vi "Action Dispatch.vi"(8 "error in (no error)":errorcluster, 10 "Actions":T1(array[cluster]), 11 "Motions in":refnum<class "Motions.lvclass">) -> (0 "error out":errorcluster, 3 "Motions out":refnum<class "Motions.lvclass">)   [LabVIEW 2016, in "Hardware.lvlib" / "Motions.lvlib" / "Motions.lvclass"]
uses:
  <userlib>/Common Components/Hardware/Abstract System/Motions/Motions/Motions.lvclass
  <userlib>/Common Components/Hardware/Abstract System/Motions/Motions/Data_Set Motion Status.ctl
  <userlib>/Common Components/Hardware/Abstract System/Motions/Motions/Data_Move.ctl
  <userlib>/Common Components/Hardware/Abstract System/Motions/Motions/Data_Index.ctl
  <userlib>/Common Components/Hardware/Abstract System/Motions/Motions/Data_Update History Dst Q.ctl
  <vilib>/Utility/error.llb/Error Cluster From Error Code.vi
  <vilib>/ErrorRing/Error Ring.xnode
  <vilib>/addons/_JKI.lib/Serialization/JSON/JKI JSON Serialization.lvlib
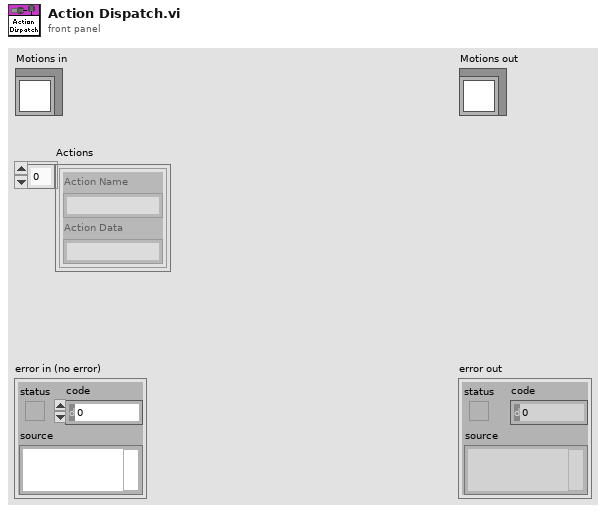
[diagram p1: front panel]
types:
  T1 = cluster{"Action Name":string, "Action Data":string}[]
  T2 = typedef "Hardware.lvlib/Motions.lvlib/Motions.lvclass/Data_Set Motion Status.ctl" = cluster{"Index":i32, "Motion Status":bool}
  T3 = typedef "Hardware.lvlib/Motions.lvlib/Motions.lvclass/Data_Move.ctl" = cluster{"Index":i32, "Destination":dbl}
  T4 = typedef "Hardware.lvlib/Motions.lvlib/Motions.lvclass/Data_Index.ctl" = cluster{"Index":i32}
  T5 = typedef "Hardware.lvlib/Motions.lvlib/Motions.lvclass/Data_Update History Dst Q.ctl" = cluster{"Index":i32, "Destination":dbl, "Mode":enum16{"Add", "Replace"}}
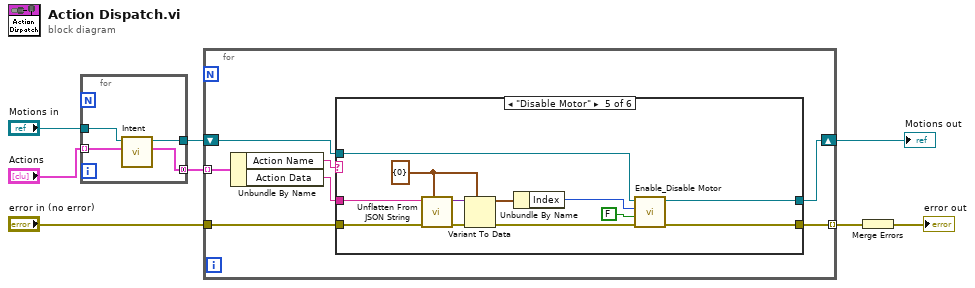
[diagram p0: block diagram]
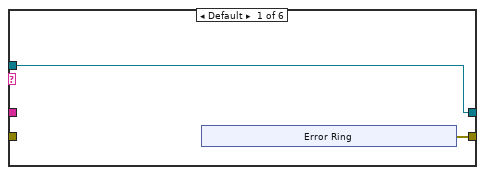
[diagram p2: hidden frame]
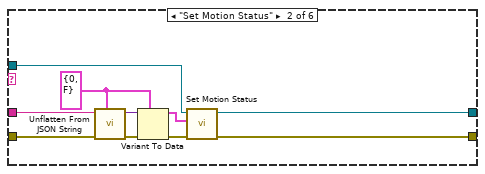
[diagram p3: hidden frame]
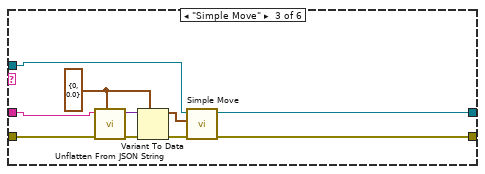
[diagram p4: hidden frame]
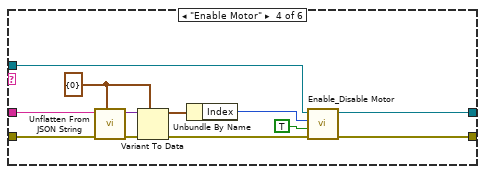
[diagram p5: hidden frame]
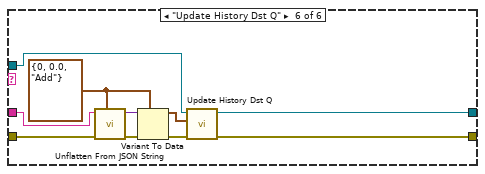
[diagram p6: hidden frame]
diagram:
  n1 = for {
    tunnel: "Actions" -> [w10] mode=indexing
    tunnel: "Motions in" -> [w12]
    tunnel: [w11] -> w2
    tunnel: [w9] -> w1 mode=concatenating
    n2 = call <userlib>:"Intent.vi"("Intent"=w10, "Motions in"=w12) -> ("Actions"=w9:T1, "Motions out"=w11:refnum<class "Motions.lvclass">)  [unwired: 7 in, 1 out]
  }
  n3 = for {
    shift-right: [w14] -> w8
    shift-left: w2 -> [w17]
    tunnel: w1 -> [w19] mode=indexing
    tunnel: "error in (no error)" -> [w15]
    tunnel: [w13] -> w6 mode=indexing
    n4 = Unbundle By Name(w19) -> ("Action Name"=w18:string, "Action Data"=w16:string)
    n5 = case shown="\"Disable Motor\"" w18 {
      tunnel: [w21 w26 w36 w50 w62 w79] -> w13
      tunnel: w17 -> [w20 w35 w40 w53 w65 w78]
      tunnel: w16 -> [_ w34 w41 w54 w66 w70]
      tunnel: w15 -> [_ w33 w43 w55 w67 w74]
      tunnel: [w20 w27 w37 w51 w63 w77] -> w14
      frame Default {
        n6 = xnode "Error Ring"() -> ("error out"=w21:errorcluster)
      }
      frame "Set Motion Status" {
        w31 = T2 {"Index"=0, "Motion Status"=FALSE} ("Set Motion Status Data cluster")
        n7 = call <vilib>:"Unflatten From JSON String.vi"("Type and Defaults"=w31, "error in (no error)"=w33, "JSON String"=w34) -> ("error out"=w30:errorcluster, "Variant"=w32:variant)  [unwired: 7 in]
        n8 = Variant To Data(error in=w30, type=w31, Variant=w32) -> (data=w28:T2, error out=w29:errorcluster)
        n9 = call <userlib>:"Set Motion Status.vi"("error in (no error)"=w29, "Set Motion Status Data cluster"=w28, "Motions in"=w35) -> ("error out"=w26:errorcluster, "Motions out"=w27:refnum<class "Motions.lvclass">)  [unwired: 7 in]
      }
      frame "Simple Move" {
        w42 = T3 {"Index"=0, "Destination"=0.0} ("Set Motion Status Data cluster")
        n10 = call <vilib>:"Unflatten From JSON String.vi"("Type and Defaults"=w42, "error in (no error)"=w43, "JSON String"=w41) -> ("error out"=w44:errorcluster, "Variant"=w45:variant)  [unwired: 7 in]
        n11 = Variant To Data(error in=w44, type=w42, Variant=w45) -> (data=w39:T3, error out=w38:errorcluster)
        n12 = call <userlib>:"Simple Move.vi"("error in (no error)"=w38, "Move Data cluster"=w39, "Motions in"=w40) -> ("error out"=w36:errorcluster, "Motions out"=w37:refnum<class "Motions.lvclass">)  [unwired: 7 in]
      }
      frame "Enable Motor" {
        w47 = T4 {"Index"=0} ("Move Data cluster")
        n13 = call <vilib>:"Unflatten From JSON String.vi"("Type and Defaults"=w47, "error in (no error)"=w55, "JSON String"=w54) -> ("error out"=w56:errorcluster, "Variant"=w57:variant)  [unwired: 7 in]
        n14 = Variant To Data(error in=w56, type=w47, Variant=w57) -> (data=w49:T4, error out=w52:errorcluster)
        n15 = Unbundle By Name(w49) -> ("Index"=w48:i32)
        n16 = call <userlib>:"Enable_Disable Motor.vi"("error in (no error)"=w52, "enable/disable"=TRUE, "Index"=w48, "Motions in"=w53) -> ("error out"=w50:errorcluster, "Motions out"=w51:refnum<class "Motions.lvclass">)  [unwired: 6 in]
      }
      frame "Disable Motor" {
        w59 = T4 {"Index"=0} ("Move Data cluster")
        n17 = call <vilib>:"Unflatten From JSON String.vi"("Type and Defaults"=w59, "error in (no error)"=w67, "JSON String"=w66) -> ("error out"=w68:errorcluster, "Variant"=w69:variant)  [unwired: 7 in]
        n18 = Variant To Data(error in=w68, type=w59, Variant=w69) -> (data=w61:T4, error out=w64:errorcluster)
        n19 = Unbundle By Name(w61) -> ("Index"=w60:i32)
        n20 = call <userlib>:"Enable_Disable Motor.vi"("error in (no error)"=w64, "enable/disable"=FALSE, "Index"=w60, "Motions in"=w65) -> ("error out"=w62:errorcluster, "Motions out"=w63:refnum<class "Motions.lvclass">)  [unwired: 6 in]
      }
      frame "Update History Dst Q" {
        w72 = T5 {"Index"=0, "Destination"=0.0, "Mode"=enum."Add"} ("Update History Dst Q Data cluster")
        n21 = call <vilib>:"Unflatten From JSON String.vi"("Type and Defaults"=w72, "error in (no error)"=w74, "JSON String"=w70) -> ("error out"=w75:errorcluster, "Variant"=w76:variant)  [unwired: 7 in]
        n22 = Variant To Data(error in=w75, type=w72, Variant=w76) -> (data=w71:T5, error out=w73:errorcluster)
        n23 = call <userlib>:"Update History Dst Q.vi"("error in (no error)"=w73, "Update History Dst Q Data cluster"=w71, "Motions in"=w78) -> ("error out"=w79:errorcluster, "Motions out"=w77:refnum<class "Motions.lvclass">)  [unwired: 7 in]
      }
    }
  }
  "Motions out" <- w8
  n24 = Merge Errors(w6) -> (→"error out":errorcluster)
